vi "Multi Points Volt to physical quantity-Waveform Data.vi"(6 "precision (6)":i16=3, 8 "error out":errorcluster, 10 "input waveform":waveform(dbl), 11 "Calibration Kb&Volts":T1) -> (0 "error out":errorcluster, 3 "output waveform":waveform(dbl))   [LabVIEW 2017, in "SQLite.lvclass"]
doc: "多点校准模块。\n2015-07-12 15:11:47\n蒋松\njiangsong@outlook.com"
uses:
  SQLite.lvclass
  Calibration Kb and Volt.ctl
  Calibration K and b Array.ctl
  Calibration K and b.ctl
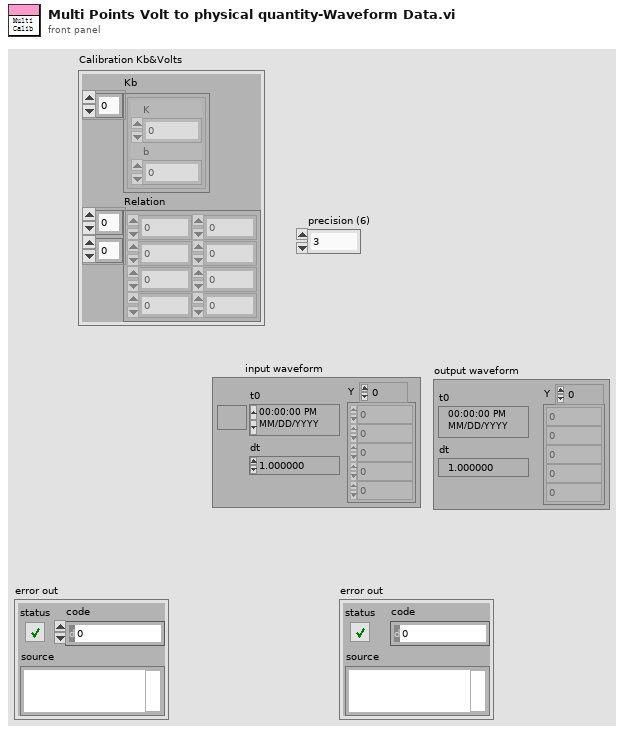
[diagram p1: front panel]
types:
  T1 = typedef "SQLite.lvclass/Calibration Kb and Volt.ctl" = cluster{"Kb":T2, "Relation":dbl[][]}
  T2 = typedef "SQLite.lvclass/Calibration K and b Array.ctl" = T3[]
  T3 = typedef "SQLite.lvclass/Calibration K and b.ctl" = cluster{"K":dbl, "b":dbl}
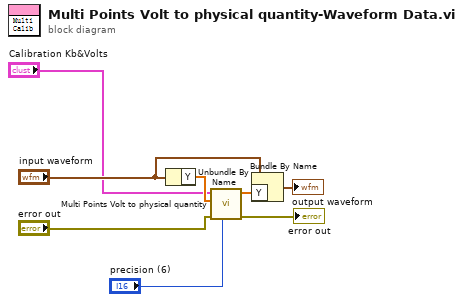
[diagram p0: block diagram]
diagram:
  n1 = Unbundle By Name("input waveform") -> ("Y"=w7:dbl[])
  n2 = call "Multi Points Volt to physical quantity.vi"("precision (6)"="precision (6)", "error out"="error out", "Real Volt"=w7, "Calibration Kb&Volts"="Calibration Kb&Volts") -> ("error out"=→"error out":errorcluster, "physical quantity"=w8:dbl[])  [unwired: 5 in, 1 out]
  n3 = Bundle By Name(cluster="input waveform", "Y"=w8) -> (→"output waveform":waveform(dbl))
